vi "Example.vi"() -> ()   [LabVIEW 2015]
uses:
  <instrlib>/Agilent N6700 Series/Agilent N6700 Series.lvlib
panel:
  in  "Channel Name (1)":string="1"
  in  "Limit (1.0 A)":dbl=-0.2 format="%.3g"
  in  "VISA resource name":refnum<visa-resource-name>="VAL_N6705B"
  in  "Delay to Measure":u32=100
  out "Voltage Measurement":dbl format="%.3f"
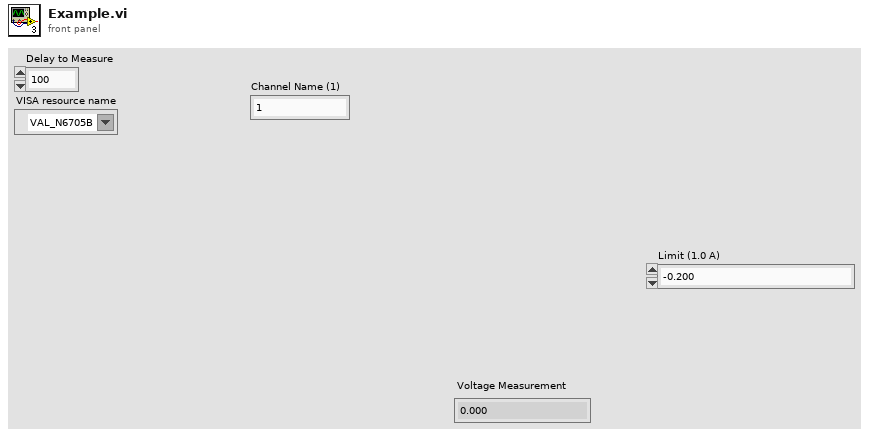
[diagram p1: front panel]
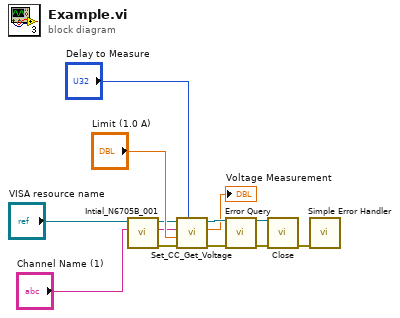
[diagram p0: block diagram]
diagram:
  n1 = call "Intial_N6705B_001.vi"("Channel Name (1) in"="Channel Name (1)", "VISA Refnum in"="VISA resource name") -> ("error out"=w1:errorcluster, "Channel Name (1) out"=w6:string, "VISA Refnum out"=w2:refnum<visa-resource-name>)  [unwired: 7 in]
  n2 = call "Set_CC_Get_Voltage.vi"("Delay to Measure"="Delay to Measure", "error in (no error)"=w1, "Limit (1.0 A)"="Limit (1.0 A)", "Channel Name (1)"=w6, "VISA Refnum in"=w2) -> ("error out"=w12:errorcluster, "Voltage Measurement"=→"Voltage Measurement":dbl, "VISA Refnum out"=w9:refnum<visa-resource-name>)  [unwired: 3 in, 1 out]
  n3 = call <instrlib>:"Error Query.vi"("VISA resource name"=w9, "error in (no error)"=w12) -> ("VISA resource name out"=w10:refnum<visa-resource-name>, "error out"=w11:errorcluster)  [unwired: 10 in, 2 out]
  n4 = call <instrlib>:"Close.vi"("VISA resource name"=w10, "error in (no error)"=w11) -> ("error out"=w13:errorcluster)  [unwired: 13 in]
  n5 = call <vilib>:"Simple Error Handler.vi"("error in (no error)"=w13) -> ()  [unwired: 4 in, 5 out]
